vi "Register Datum.vi"(8 "error in (no error)":errorcluster, 10 "Full Factory in":refnum<class "Full Factory.lvclass">, 11 "UI Controller in":refnum<class "UI Controller.lvclass">) -> (0 "error out":errorcluster, 3 "UI Controller out":refnum<class "UI Controller.lvclass">)   [LabVIEW 2020, in "UI Controller.lvlib" / "Full Factory.lvclass"]
uses:
  Full Factory.lvclass
  UI Controller/UI Controller.lvclass
panel:
  # "NOTICE -- YOU MUST LEAVE THIS NOTICE IN PLACE.\n\nCopyright (c) 2017, LIANG LIU Shawn.Liu.cn@gmail.com\nAll rights reserved.\n\nRedistribution and use in source and binary forms, with or without modification, are permitted provided that the following conditions are met:\n-Redistributions of source code must retain the above copyright notice, this list of conditions and the following disclaimer.\n-Redistributions in binary form must reproduce the above copyright notice, this list of conditions and the following disclaimer in the documentation and/or other materials provided with the distribution.\n-Neither the name of the eLp nor the names of its contributors may be used to endorse or promote products derived from this software without specific prior written permission.\n\nTHIS SOFTWARE IS PROVIDED BY THE COPYRIGHT HOLDERS AND CONTRIBUTORS \"AS IS\" AND ANY EXPRESS OR IMPLIED WARRANTIES, INCLUDING, BUT NOT LIMITED TO, THE IMPLIED WARRANTIES OF MERCHANTABILITY AND FITNESS FOR A PARTICULAR PURPOSE ARE DISCLAIMED. IN NO EVENT SHALL THE COPYRIGHT HOLDER OR CONTRIBUTORS BE LIABLE FOR ANY DIRECT, INDIRECT, INCIDENTAL, SPECIAL, EXEMPLARY, OR CONSEQUENTIAL DAMAGES (INCLUDING, BUT NOT LIMITED TO, PROCUREMENT OF SUBSTITUTE GOODS OR SERVICES; LOSS OF USE, DATA, OR PROFITS; OR BUSINESS INTERRUPTION) HOWEVER CAUSED AND ON ANY THEORY OF LIABILITY, WHETHER IN CONTRACT, STRICT LIABILITY, OR TORT (INCLUDING NEGLIGENCE OR OTHERWISE) ARISING IN ANY WAY OUT OF THE USE OF THIS SOFTWARE, EVEN IF ADVISED OF THE POSSIBILITY OF SUCH DAMAGE."
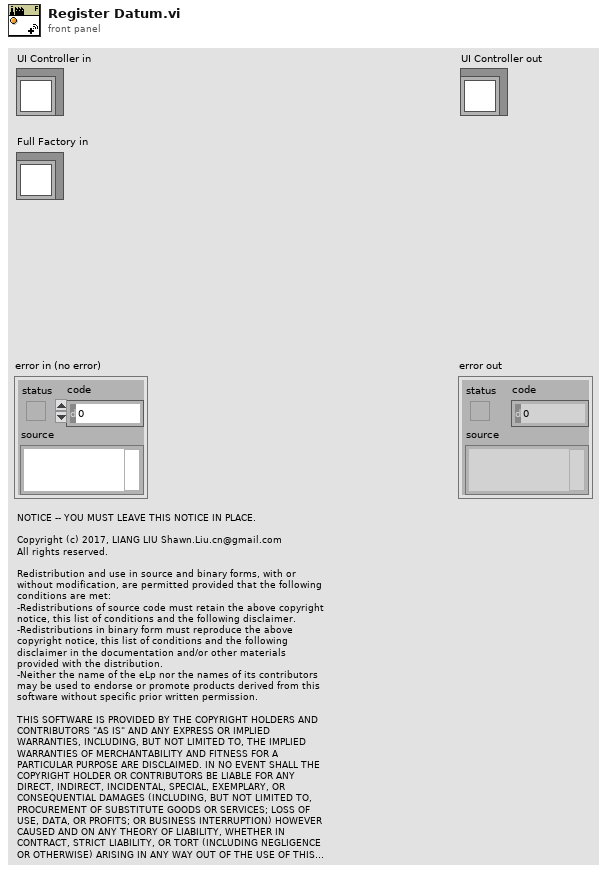
[diagram p1: front panel]
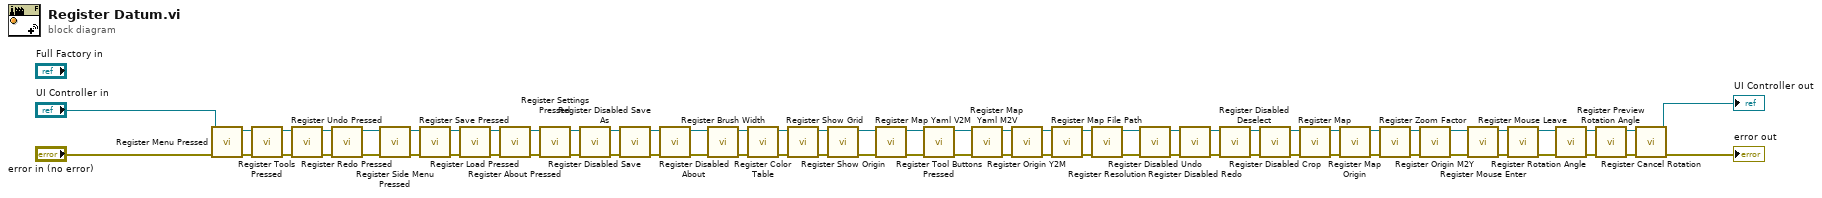
[diagram p0: block diagram]
diagram:
  n1 = call "Register Menu Pressed.vi"("error in (no error)"="error in (no error)", "UI Controller in"="UI Controller in") -> ("error out"=w67:errorcluster, "UI Controller out"=w68:refnum<class "UI Controller.lvclass">)  [unwired: 8 in]
  n2 = call "Register Tools Pressed.vi"("error in (no error)"=w67, "UI Controller in"=w68) -> ("error out"=w50:errorcluster, "UI Controller out"=w51:refnum<class "UI Controller.lvclass">)  [unwired: 8 in]
  n3 = call "Register Undo Pressed.vi"("error in (no error)"=w50, "UI Controller in"=w51) -> ("error out"=w48:errorcluster, "UI Controller out"=w49:refnum<class "UI Controller.lvclass">)  [unwired: 8 in]
  n4 = call "Register Redo Pressed.vi"("error in (no error)"=w48, "UI Controller in"=w49) -> ("error out"=w12:errorcluster, "UI Controller out"=w13:refnum<class "UI Controller.lvclass">)  [unwired: 8 in]
  n5 = call "Register Side Menu Pressed.vi"("error in (no error)"=w12, "UI Controller in"=w13) -> ("error out"=w65:errorcluster, "UI Controller out"=w66:refnum<class "UI Controller.lvclass">)  [unwired: 8 in]
  n6 = call "Register Save Pressed.vi"("error in (no error)"=w65, "UI Controller in"=w66) -> ("error out"=w63:errorcluster, "UI Controller out"=w64:refnum<class "UI Controller.lvclass">)  [unwired: 8 in]
  n7 = call "Register Load Pressed.vi"("error in (no error)"=w63, "UI Controller in"=w64) -> ("error out"=w61:errorcluster, "UI Controller out"=w62:refnum<class "UI Controller.lvclass">)  [unwired: 8 in]
  n8 = call "Register About Pressed.vi"("error in (no error)"=w61, "UI Controller in"=w62) -> ("error out"=w59:errorcluster, "UI Controller out"=w60:refnum<class "UI Controller.lvclass">)  [unwired: 8 in]
  n9 = call "Register Settings Pressed.vi"("error in (no error)"=w59, "UI Controller in"=w60) -> ("error out"=w57:errorcluster, "UI Controller out"=w58:refnum<class "UI Controller.lvclass">)  [unwired: 8 in]
  n10 = call "Register Disabled Save.vi"("error in (no error)"=w57, "UI Controller in"=w58) -> ("error out"=w69:errorcluster, "UI Controller out"=w70:refnum<class "UI Controller.lvclass">)  [unwired: 8 in]
  n11 = call "Register Disabled Save As.vi"("error in (no error)"=w69, "UI Controller in"=w70) -> ("error out"=w55:errorcluster, "UI Controller out"=w56:refnum<class "UI Controller.lvclass">)  [unwired: 8 in]
  n12 = call "Register Disabled About.vi"("error in (no error)"=w55, "UI Controller in"=w56) -> ("error out"=w41:errorcluster, "UI Controller out"=w42:refnum<class "UI Controller.lvclass">)  [unwired: 8 in]
  n13 = call "Register Brush Width.vi"("error in (no error)"=w41, "UI Controller in"=w42) -> ("error out"=w39:errorcluster, "UI Controller out"=w40:refnum<class "UI Controller.lvclass">)  [unwired: 8 in]
  n14 = call "Register Color Table.vi"("error in (no error)"=w39, "UI Controller in"=w40) -> ("error out"=w38:errorcluster, "UI Controller out"=w28:refnum<class "UI Controller.lvclass">)  [unwired: 8 in]
  n15 = call "Register Show Grid.vi"("error in (no error)"=w38, "UI Controller in"=w28) -> ("error out"=w2:errorcluster, "UI Controller out"=w27:refnum<class "UI Controller.lvclass">)  [unwired: 8 in]
  n16 = call "Register Show Origin.vi"("error in (no error)"=w2, "UI Controller in"=w27) -> ("error out"=w1:errorcluster, "UI Controller out"=w3:refnum<class "UI Controller.lvclass">)  [unwired: 8 in]
  n17 = call "Register Map Yaml V2M.vi"("error in (no error)"=w1, "UI Controller in"=w3) -> ("error out"=w36:errorcluster, "UI Controller out"=w37:refnum<class "UI Controller.lvclass">)  [unwired: 8 in]
  n18 = call "Register Tool Buttons Pressed.vi"("error in (no error)"=w36, "UI Controller in"=w37) -> ("error out"=w34:errorcluster, "UI Controller out"=w35:refnum<class "UI Controller.lvclass">)  [unwired: 8 in]
  n19 = call "Register Map Yaml M2V.vi"("error in (no error)"=w34, "UI Controller in"=w35) -> ("error out"=w33:errorcluster, "UI Controller out"=w18:refnum<class "UI Controller.lvclass">)  [unwired: 8 in]
  n20 = call "Register Origin Y2M.vi"("error in (no error)"=w33, "UI Controller in"=w18) -> ("error out"=w19:errorcluster, "UI Controller out"=w17:refnum<class "UI Controller.lvclass">)  [unwired: 8 in]
  n21 = call "Register Map File Path.vi"("error in (no error)"=w19, "UI Controller in"=w17) -> ("error out"=w44:errorcluster, "UI Controller out"=w43:refnum<class "UI Controller.lvclass">)  [unwired: 8 in]
  n22 = call "Register Resolution.vi"("error in (no error)"=w44, "UI Controller in"=w43) -> ("error out"=w10:errorcluster, "UI Controller out"=w11:refnum<class "UI Controller.lvclass">)  [unwired: 8 in]
  n23 = call "Register Disabled Undo.vi"("error in (no error)"=w10, "UI Controller in"=w11) -> ("error out"=w53:errorcluster, "UI Controller out"=w52:refnum<class "UI Controller.lvclass">)  [unwired: 8 in]
  n24 = call "Register Disabled Redo.vi"("error in (no error)"=w53, "UI Controller in"=w52) -> ("error out"=w8:errorcluster, "UI Controller out"=w9:refnum<class "UI Controller.lvclass">)  [unwired: 8 in]
  n25 = call "Register Disabled Deselect.vi"("error in (no error)"=w8, "UI Controller in"=w9) -> ("error out"=w6:errorcluster, "UI Controller out"=w7:refnum<class "UI Controller.lvclass">)  [unwired: 8 in]
  n26 = call "Register Disabled Crop.vi"("error in (no error)"=w6, "UI Controller in"=w7) -> ("error out"=w4:errorcluster, "UI Controller out"=w5:refnum<class "UI Controller.lvclass">)  [unwired: 8 in]
  n27 = call "Register Map.vi"("error in (no error)"=w4, "UI Controller in"=w5) -> ("error out"=w54:errorcluster, "UI Controller out"=w46:refnum<class "UI Controller.lvclass">)  [unwired: 8 in]
  n28 = call "Register Map Origin.vi"("error in (no error)"=w54, "UI Controller in"=w46) -> ("error out"=w47:errorcluster, "UI Controller out"=w45:refnum<class "UI Controller.lvclass">)  [unwired: 8 in]
  n29 = call "Register Zoom Factor.vi"("error in (no error)"=w47, "UI Controller in"=w45) -> ("error out"=w32:errorcluster, "UI Controller out"=w15:refnum<class "UI Controller.lvclass">)  [unwired: 8 in]
  n30 = call "Register Origin M2Y.vi"("error in (no error)"=w32, "UI Controller in"=w15) -> ("error out"=w16:errorcluster, "UI Controller out"=w14:refnum<class "UI Controller.lvclass">)  [unwired: 8 in]
  n31 = call "Register Mouse Enter.vi"("error in (no error)"=w16, "UI Controller in"=w14) -> ("error out"=w31:errorcluster, "UI Controller out"=w29:refnum<class "UI Controller.lvclass">)  [unwired: 8 in]
  n32 = call "Register Mouse Leave.vi"("error in (no error)"=w31, "UI Controller in"=w29) -> ("error out"=w30:errorcluster, "UI Controller out"=w25:refnum<class "UI Controller.lvclass">)  [unwired: 8 in]
  n33 = call "Register Rotation Angle.vi"("error in (no error)"=w30, "UI Controller in"=w25) -> ("error out"=w26:errorcluster, "UI Controller out"=w23:refnum<class "UI Controller.lvclass">)  [unwired: 8 in]
  n34 = call "Register Preview Rotation Angle.vi"("error in (no error)"=w26, "UI Controller in"=w23) -> ("error out"=w24:errorcluster, "UI Controller out"=w21:refnum<class "UI Controller.lvclass">)  [unwired: 8 in]
  n35 = call "Register Cancel Rotation.vi"("error in (no error)"=w24, "UI Controller in"=w21) -> ("error out"=→"error out":errorcluster, "UI Controller out"=→"UI Controller out":refnum<class "UI Controller.lvclass">)  [unwired: 8 in]
